vi "first_coma_to_period.vi"(11 "string_in":string) -> (3 "string_out":string)   [LabVIEW 2019]
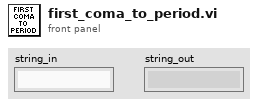
[diagram p1: front panel]
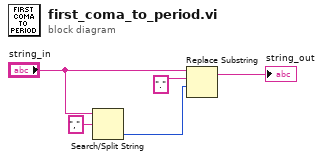
[diagram p0: block diagram]
diagram:
  n1 = Search/Split String(string="string_in", search string/char (-)=",") -> (offset of match=w3:i32)  [unwired: 1 in, 2 out]
  n2 = Replace Substring(3:w3, 4:"." ("substring (\"\")"), 5:"string_in") -> (1:→"string_out":string)  [unwired: 1 in, 1 out]
